vi "Scan Nodes Wrapper.vi"(8 "error in (no error)":errorcluster, 9 "timeout_ms":u64=2000, 10 "Key Filter":string="*", 11 "Reader Handle":u64) -> (0 "error out":errorcluster, 2 "Length":i32, 3 "buffer_out":string)   [LabVIEW 2021, in "Zenoh.lvclass"]
uses:
  Zenoh.lvclass
  Zenoh.lvclass/Zenoh.ctl
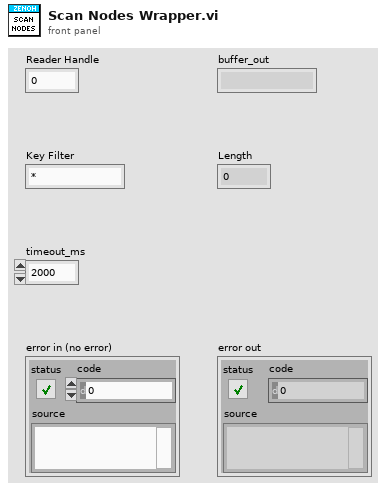
[diagram p1: front panel]
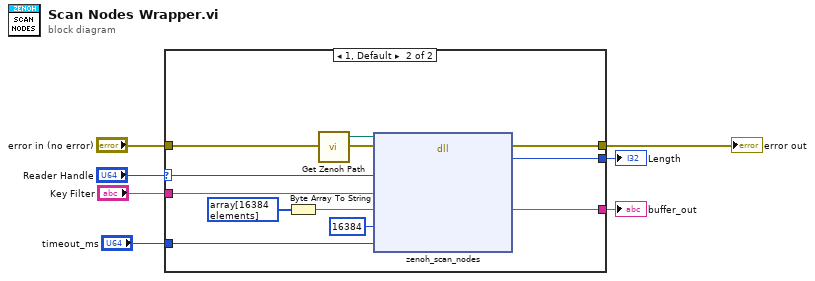
[diagram p0: block diagram]
diagram:
  n1 = case shown="1, Default" "Reader Handle" {
    selector: "Reader Handle" -> [_ w18]
    tunnel: [w8 w16] -> w7
    tunnel: "error in (no error)" -> [w8 w19]
    tunnel: [_ w11] -> w2
    tunnel: "Key Filter" -> [_ w13]
    tunnel: "timeout_ms" -> [_ w10]
    tunnel: [_ w9] -> w1
    frame 0 {
    }
    frame 1, Default {
      n2 = Byte Array To String(unsigned byte array=u8[] array[16384 elements] ("Buffer in")) -> (string=w14:string)
      n3 = call "Get Zenoh Path.vi"() -> ("Library Path"=w17:path)  [unwired: 4 in]
      n4 = dll-call lib="C:/Program Files/CIF_Foundation/Libraries/zenoh_lv_wrapper.dll" fn="zenoh_scan_nodes"(path in=w17, error in=w19, "session_ptr"=w18, "key_filter"=w13, "buffer_out"=w14, "max_buffer_size"=16384, "timeout_ms"=w10) -> (error out=w16:errorcluster, "return type"=w9:i32, "buffer_out"=w11:string)  [unwired: 5 in, 1 out]
    }
  }
  "error out" <- w7
  "buffer_out" <- w2
  "Length" <- w1
